vi "SpectrumCursor_readGroupIndices.vi"(1 "first 4 letters\nfrom cursor\nname":string, 2 "Cursor List":T1(array[cluster])) -> (0 "cursors\nindeces":i32[](array[numeric]))   [LabVIEW 2010]
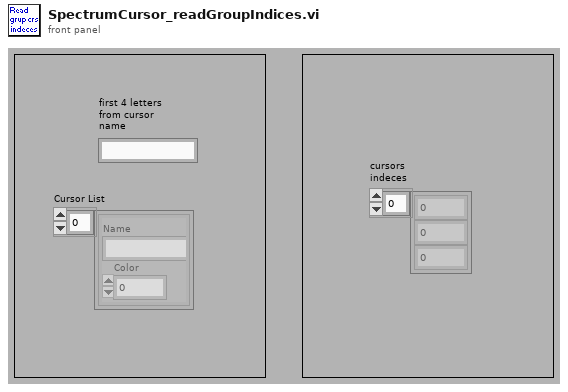
[diagram p1: front panel]
types:
  T1 = cluster{"Name":string, "Color":u32, "Style":u8, "Point Style":u8, "Name Visible":bool, "Allow Drag":bool, "Cursor Mode":u32, "Plot":i32, "Index":i32, "Position":cluster{"X":dbl, "Y":dbl}, "X Scale":u32, "Y Scale":u32, "Watch Plots":i32[], "Watch All Plots":bool, "Plot Area":i32, "Label Offset":cluster{"X":dbl, "Y":dbl}}[]
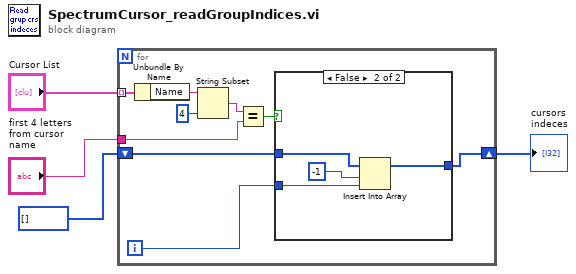
[diagram p0: block diagram]
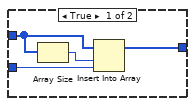
[diagram p2: hidden frame]
diagram:
  n1 = for {
    tunnel: "Cursor List" -> [w13] mode=indexing
    tunnel: "first 4 letters\nfrom cursor\nname" -> [w7]
    shift-right: [w6] -> w1
    shift-left: i32[] [] ("cursors\nindeces 2") -> [w5]
    i -> [w8]
    n2 = Unbundle By Name(w13) -> ("Name"=w12:string)
    n3 = String Subset(string=w12, length (rest)=4 ("length (rest)")) -> (substring=w10:string)  [unwired: 1 in]
    n4 = Equal?(x=w10, y=w7) -> (x = y?=w9:bool)
    n5 = case shown="False" w9 {
      tunnel: w8 -> [w17 w21]
      tunnel: [w16 w20] -> w6
      tunnel: w5 -> [w14 w19]
      frame True {
        n6 = Array Size(array=w14) -> (size(s)=w15:i32)
        n7 = Insert Into Array(array=w14, index=w15, new element=w17) -> (w16:i32[])
      }
      frame False {
        n8 = Insert Into Array(array=w19, index=-1, new element=w21) -> (w20:i32[])
      }
    }
  }
  "cursors\nindeces" <- w1
